vi "_CheckUserLegal.vi"(8 "error in (no error)":errorcluster, 11 "Username":string) -> (0 "error out":errorcluster, 2 "Legal?":bool)   [LabVIEW 2017, in "Login-UI.lvlib"]
uses:
  Login-UI.lvlib
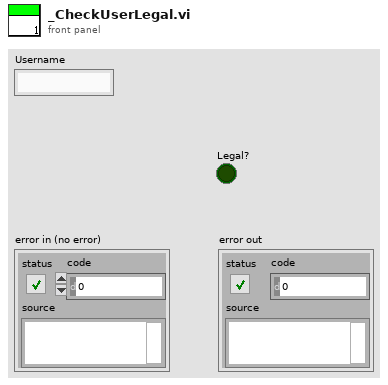
[diagram p1: front panel]
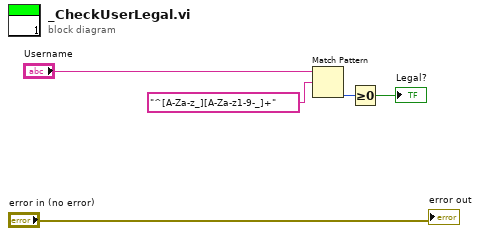
[diagram p0: block diagram]
diagram:
  n1 = Match Pattern(string="Username", regular expression="^[A-Za-z_][A-Za-z1-9-_]+") -> (offset past match=w4:i32)  [unwired: 1 in, 3 out]
  n2 = Greater Or Equal To 0?(x=w4) -> (x >= 0?=→"Legal?":bool)
  "error out" <- "error in (no error)"
